vi "Write Sensor Enqueuers.vi"(8 "error in (no error)":errorcluster, 10 "Sensor Enqueuers":refnum<class "Message Enqueuer.lvclass">[](array[class]), 11 "DemoMain in":refnum<class "DemoMain.lvclass">) -> (0 "error out":errorcluster, 3 "DemoMain out":refnum<class "DemoMain.lvclass">)   [LabVIEW 2012, in "Win8uiDemo.lvlib" / "DemoMain.lvclass"]
uses:
  DemoMain.lvclass
  <vilib>/ActorFramework/Message Enqueuer/Message Enqueuer.lvclass
  DemoMain.lvclass/DemoMain.ctl
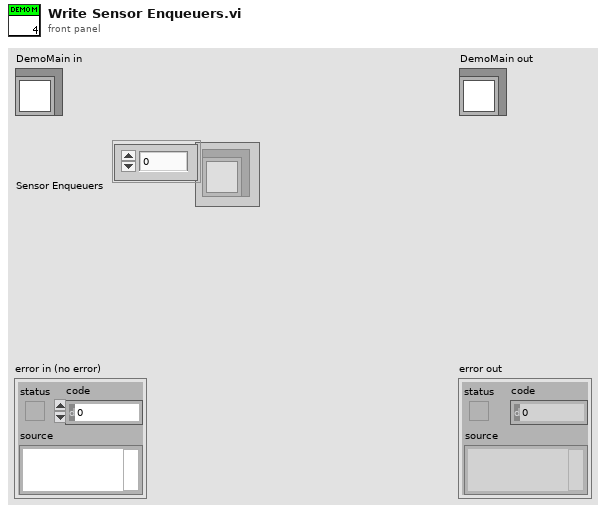
[diagram p1: front panel]
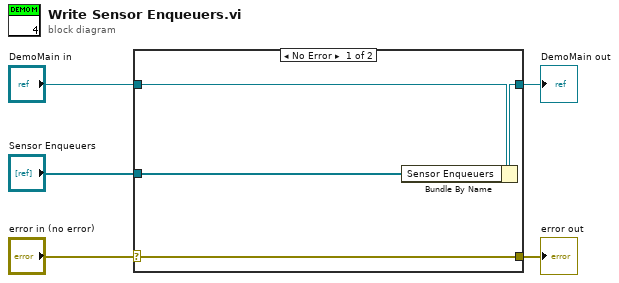
[diagram p0: block diagram]
diagram:
  n1 = case shown="No Error" "error in (no error)" {
    selector: "error in (no error)" -> [w9 w10]
    tunnel: [w9 w10] -> w4
    tunnel: [w7 w11] -> w2
    tunnel: "DemoMain in" -> [w8 w11]
    tunnel: "Sensor Enqueuers" -> [w6 _]
    frame No Error {
      n2 = Bundle By Name(cluster=w8, "Sensor Enqueuers"=w6) -> (w7:refnum<class "DemoMain.lvclass">)
    }
    frame Error {
    }
  }
  "error out" <- w4
  "DemoMain out" <- w2
